vi "Save DB Images.vi"(1 "Images to Keep":dbl=60.0, 2 "Time Interval (s)":dbl=1.0, 3 "Image":T1) -> ()   [LabVIEW 2014]
uses:
  <vilib>/vision/Image Controls.llb/IMAQ Image.ctl
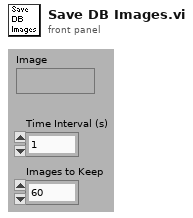
[diagram p1: front panel]
types:
  T1 = typedef "IMAQ Image.ctl" = refnum<image>
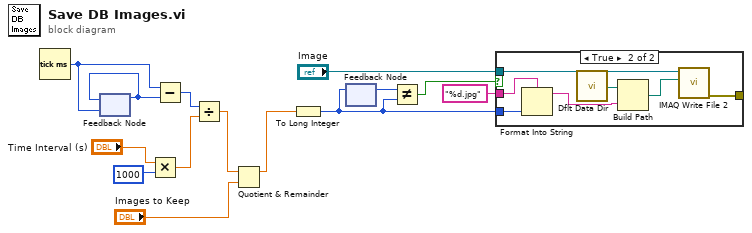
[diagram p0: block diagram]
diagram:
  n1 = Tick Count (ms)() -> (millisecond timer value=w9:u32)
  n2 = feedback #1(w9) -> (w8:u32)
  n3 = feedback-in #1(w8) -> ()
  n4 = Multiply(x="Time Interval (s)", y=1000) -> (x*y=w5:dbl)
  n5 = Subtract(x=w9, y=w8) -> (x-y=w11:u32)
  n6 = Divide(x=w11, y=w5) -> (x/y=w2:dbl)
  n7 = Quotient & Remainder(x=w2, y="Images to Keep") -> (x-y*floor(x/y)=w1:dbl)  [unwired: 1 out]
  n8 = To Long Integer(number=w1) -> (32bit integer=w3:i32)
  n9 = feedback-in #2(w3) -> ()
  n10 = feedback #2() -> (w13:i32)  [unwired: 1 out]
  n11 = Not Equal?(x=w13, y=w3) -> (x != y?=w14:bool)
  n12 = case shown="True" w14 {
    tunnel: "Image" -> [_ w21]
    tunnel: [_ w18] -> _
    tunnel: "%d.jpg" ("format string") -> [_ w15]
    tunnel: w3 -> [_ w16]
    frame False {
    }
    frame True {
      n13 = Format Into String(format string=w15, w16) -> (resulting string=w17:string)  [unwired: 2 in, 1 out]
      n14 = call <vilib>:"Dflt Data Dir.vi"() -> ("App:Default Data Directory"=w20:path)
      n15 = Build Path(base path=w20, name or relative path=w17) -> (appended path=w19:path)
      n16 = call-poly "IMAQ Write File 2"("File Path"=w19, "Image"=w21) -> ("error out"=w18:errorcluster)  [unwired: 3 in, 6 out]
    }
  }
